vi "G#SubTemplateG3_GetClassAttributesToModify.vi"(0 "reference in":refnum<class "G#SubTemplateG3.lvclass">, 3 "timeout in ms (-1)":i32=-1, 5 "error in (no error)":errorcluster) -> (14 "reference out":refnum<class "G#SubTemplateG3.lvclass">, 15 "class attributes ref":T3, 16 "class attributes":T1, 17 "timeout":bool, 18 "created new":bool, 19 "error out":errorcluster)   [LabVIEW 2020, in "G#SubTemplateG3.lvclass"]
doc: "This VI returns the attributes associated with this class or subclass object reference and places a lock on the object.\n\nIf the object is currently locked for modification by another method, 'Timeout' specifies how long the VI should wait to receive access to the object. The default value waits until the object becomes available.\n\nYou must use this class SetModifiedAttributes VI to set the object's data and release the lock."
uses:
  <vilib>/addons/_AddQ/G#Templates/G#SubTemplateG3/G#SubTemplateG3.lvclass
  <vilib>/addons/_AddQ/G#Templates/G#SubTemplateG3/utils/ClassAttributesRef.ctl
  <vilib>/addons/_AddQ/G#Templates/G#SubTemplateG3/protected/ClassAttributes.ctl
  <vilib>/addons/_AddQ/G#Templates/G#BaseTemplateG3/protected/ClassAttributes.ctl
  <vilib>/addons/_AddQ/G#Templates/G#SubTemplateG3/G#SubTemplateG3.lvclass/G#SubTemplateG3.ctl
  <vilib>/addons/_AddQ/G#Templates/G#BaseTemplateG3/G#BaseTemplateG3.lvclass
  C:/Program Files (x86)/National Instruments/LabVIEW 2020/vi.lib/addons/_AddQ/G#Templates/G#BaseTemplateG3/G#BaseTemplateG3.lvclass
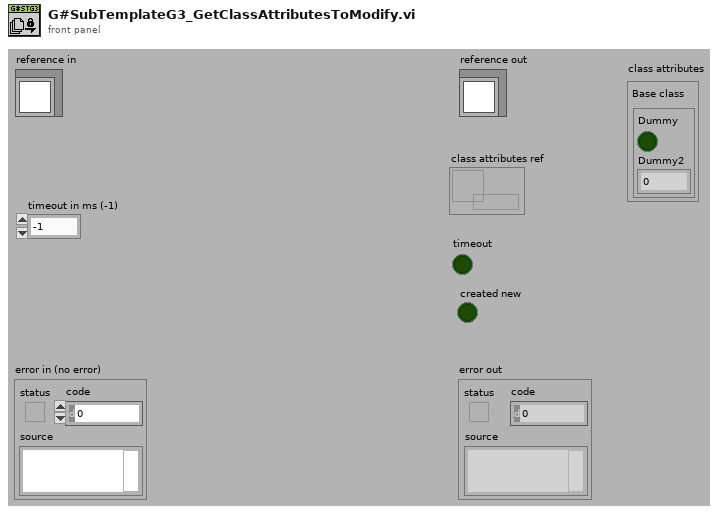
[diagram p1: front panel]
types:
  T1 = typedef "G#SubTemplateG3.lvclass/ClassAttributes.ctl" = cluster{"Base class":T2}
  T2 = typedef "G#BaseTemplateG3.lvclass/ClassAttributes.ctl" = cluster{"Dummy":bool, "Dummy2":dbl}
  T3 = typedef "G#SubTemplateG3.lvclass/ClassAttributesRef.ctl" = refnum<data-value>
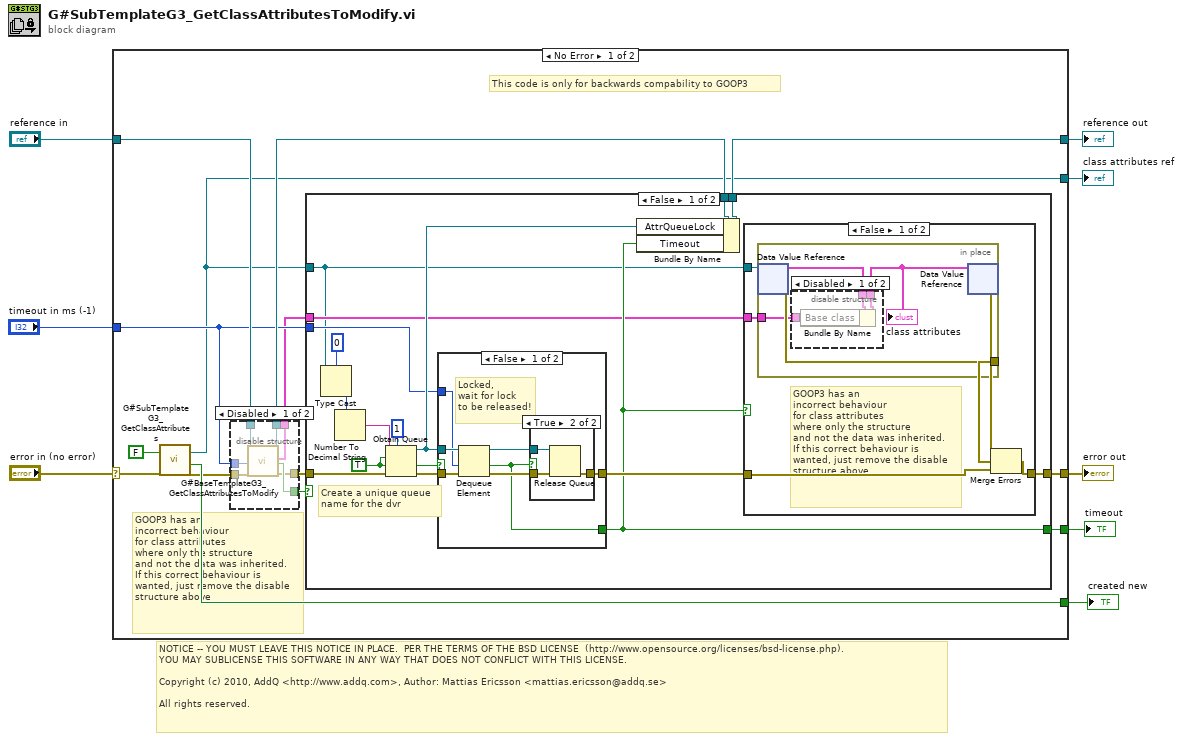
[diagram p0: block diagram]
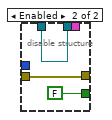
[diagram p2: hidden frame]
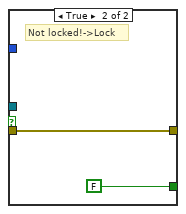
[diagram p4: hidden frame]
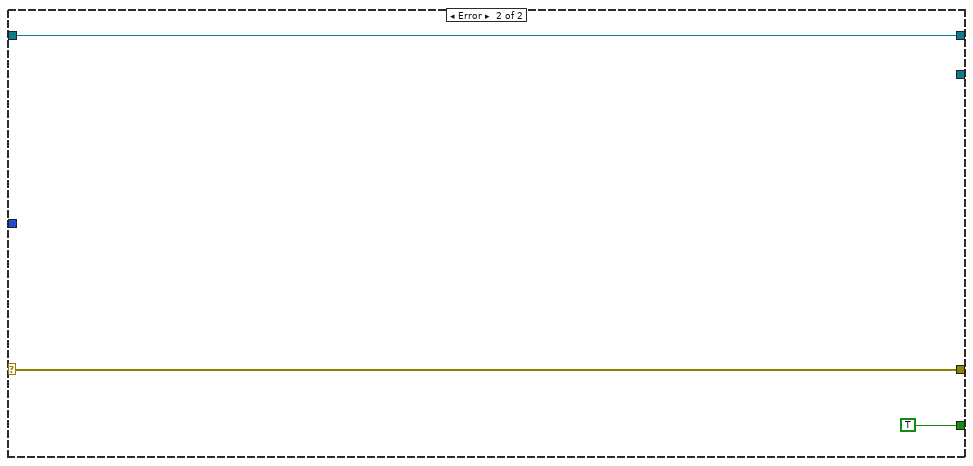
[diagram p8: hidden frame]
diagram:
  # "NOTICE -- YOU MUST LEAVE THIS NOTICE IN PLACE.  PER THE TERMS OF THE BSD LICENSE  (http://www.opensource.org/licenses/bsd-license.php).\nYOU MAY SUBLICENSE THIS SOFTWARE IN ANY WAY THAT DOES NOT CONFLICT WITH THIS LICENSE.\n\nCopyright (c) 2010, AddQ <http://www.addq.com>, Author: Mattias Ericsson <mattias.ericsson@addq.se>\n\nAll rights reserved."
  n1 = case shown="No Error" "error in (no error)" {
    selector: "error in (no error)" -> [w9 w83]
    tunnel: [w22 w83] -> w7
    tunnel: [w17 w82] -> w5
    tunnel: "reference in" -> [w20 w82]
    tunnel: [w13 _] -> w4
    tunnel: "timeout in ms (-1)" -> [w18 _]
    tunnel: [w16 TRUE ("status")] -> w2
    tunnel: [w11 _] -> w1
    frame No Error {
      # "GOOP3 has an\nincorrect behaviour\nfor class attributes\nwhere only the structure\nand not the data was inherited.\nIf this correct behaviour is\nwanted, just remove the disable\nstructure above"
      # "This code is only for backwards compability to GOOP3"
      n2 = call <vilib>:"G#SubTemplateG3_GetClassAttributes.vi"("return data? (T)"=FALSE ("return data"), "error in (no error)"=w9) -> ("class attributes ref"=w13:T3, "created new"=w11:bool, "error out"=w10:errorcluster)  [unwired: 13 in, 2 out]
      n3 = disable-structure shown="Disabled" {
        disable-tunnel: w20 -> [w29 w31]
        disable-tunnel: [w28 w31] -> w19
        disable-tunnel: w18 -> [w27 _]
        disable-tunnel: [w26 _] -> w15
        disable-tunnel: [w25 FALSE ("timeout")] -> w14
        disable-tunnel: [w24 w32] -> w12
        disable-tunnel: w10 -> [w23 w32]
        frame Disabled {
          n4 = call <vilib>:"G#BaseTemplateG3_GetClassAttributesToModify.vi"("reference in"=w29, "timeout in ms (-1)"=w27, "error in (no error)"=w23) -> ("reference out"=w28:refnum<class "G#SubTemplateG3.lvclass">, "class attributes"=w26:T2, "timeout"=w25:bool, "error out"=w24:errorcluster)  [unwired: 11 in, 2 out]
        }
        frame Enabled {
        }
      }
      n5 = case shown="False" w14 {
        selector: w14 -> [_ w79]
        tunnel: [w49 w78] -> w22
        tunnel: w12 -> [w41 w78]
        tunnel: w19 -> [w38 w80]
        tunnel: w18 -> [w37 _]
        tunnel: [w36 w80] -> w17
        tunnel: [w35 w79] -> w16
        tunnel: w15 -> [w34 _]
        tunnel: w13 -> [w33 _]
        frame False {
          w47 = TRUE ("create if not found? (T)")
          # "Create a unique queue\nname for the dvr"
          n6 = Type Cast(type=u32 0, x=w33) -> (*(type *) &x=w40:u32)
          n7 = Number To Decimal String(number=w40) -> (decimal integer string=w48:string)  [unwired: 1 in]
          n8 = Obtain Queue(max queue size (-1, unlimited)=1, name (unnamed)=w48, element data type=w47, create if not found? (T)=w47, error in (no error)=w41) -> (queue out=w42:refnum<queue>, created new?=w44:bool, error out=w45:errorcluster)
          n9 = case shown="False" w44 {
            tunnel: w45 -> [w54 w61]
            tunnel: [w53 w61] -> w43
            tunnel: w42 -> [w56 _]
            tunnel: w37 -> [w55 _]
            tunnel: [w50 FALSE ("status")] -> w35
            frame False {
              # "Locked,\nwait for lock\nto be released!"
              n10 = Dequeue Element(queue=w56, timeout in ms (-1)=w55, error in (no error)=w54) -> (queue out=w51:refnum<queue>, timed out?=w50:bool, error out=w52:errorcluster)  [unwired: 1 out]
              n11 = case shown="True" w50 {
                tunnel: [w57 w60] -> w53
                tunnel: w52 -> [w57 w59]
                tunnel: w51 -> [_ w58]
                frame False {
                }
                frame True {
                  n12 = Release Queue(queue=w58, error in (no error)=w59) -> (error out=w60:errorcluster)  [unwired: 1 in, 2 out]
                }
              }
            }
            frame True {
              # "Not locked!->Lock"
            }
          }
          n13 = Bundle By Name(cluster=w38, "AttrQueueLock"=w42, "Timeout"=w35) -> (w36:refnum<class "G#SubTemplateG3.lvclass">)
          n14 = case shown="False" w35 {
            tunnel: w33 -> [w68 _]
            tunnel: w43 -> [w67 w77]
            tunnel: [w64 w77] -> w49
            tunnel: w34 -> [w63 _]
            frame False {
              # "GOOP3 has an\nincorrect behaviour\nfor class attributes\nwhere only the structure\nand not the data was inherited.\nIf this correct behaviour is\nwanted, just remove the disable\nstructure above"
              n15 = in-place {
                in-place-border: [w70] -> w66
                in-place-border: w63 -> [w69]
                n16 = in-place-dvr #1(w68) -> (w72:T1, w70:errorcluster)
                n17 = disable-structure shown="Disabled" {
                  disable-tunnel: w72 -> [w75 w76]
                  disable-tunnel: [w74 w76] -> w71
                  disable-tunnel: w69 -> [w73 _]
                  frame Disabled {
                    n18 = Bundle By Name(cluster=w75, "Base class"=w73) -> (w74:T1)
                  }
                  frame Enabled {
                  }
                }
                "class attributes" <- w71
                n19 = in-place-dvr #1(w71) -> (w65:errorcluster)  [unwired: 1 out]
              }
              n20 = Merge Errors(w65, w66, w67) -> (w64:errorcluster)
            }
            frame True {
              # "Timeout"
            }
          }
        }
        frame True {
        }
      }
    }
    frame Error {
    }
  }
  "error out" <- w7
  "reference out" <- w5
  "class attributes ref" <- w4
  "timeout" <- w2
  "created new" <- w1
